vi "Append image and delete if possible.vi"(0 "report in":refnum<class "NI_Standard Report.lvclass">, 1 "alignment (default)":T1, 5 "path to image":path, 11 "error in (no error)":errorcluster, 12 "caption or alternative string":string, 13 "MS Office parameters":T2) -> (4 "report out":refnum<class "NI_Standard Report.lvclass">, 8 "start out (Word)":i32, 10 "end out (Word)":i32, 15 "error out":errorcluster)   [LabVIEW 2017, in "NI_Standard Report.lvclass"]
uses:
  <vilib>/Utility/NIReport.llb/Standard Report/NI_Standard Report.lvclass
  e:/builds/penguin/labview/branches/2017/dev/dist/vi.lib/Utility/NIReport.llb/NI_report.lvclass
  <vilib>/Utility/NIReport.llb/HTML Report Image Alignment.ctl
  <vilib>/Utility/NIReport.llb/NI_report.lvclass
  <vilib>/Utility/NIReport.llb/NI_ReportGenerationCore.lvlib
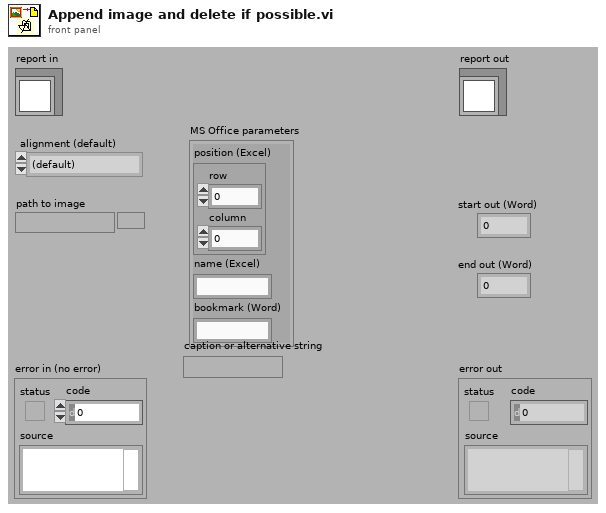
[diagram p1: front panel]
types:
  T1 = typedef "NI_ReportGenerationCore.lvlib/HTML Report Image Alignment.ctl" = enum16{"(default)", "LEFT", "RIGHT", "TOP", "TEXTTOP", "MIDDLE", "ABSMIDDLE", "BASELINE", "BOTTOM", "ABSBOTTOM"}
  T2 = cluster{"position (Excel)":cluster{"row":i32, "column":i32}, "name (Excel)":string, "bookmark (Word)":string}
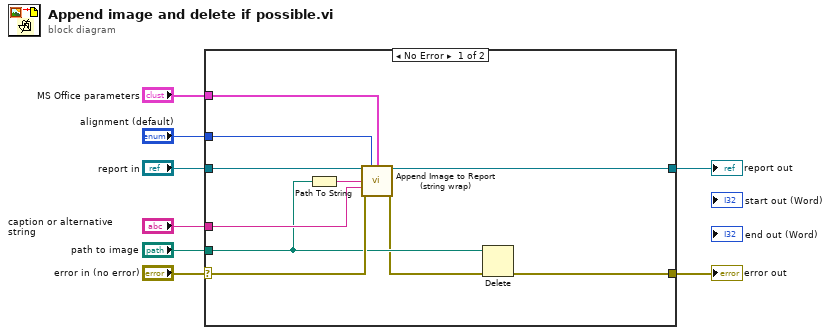
[diagram p0: block diagram]
diagram:
  n1 = case shown="No Error" "error in (no error)" {
    selector: "error in (no error)" -> [w17 w20]
    tunnel: [w9 w20] -> w7
    tunnel: [w10 w19] -> w5
    tunnel: "report in" -> [w11 w19]
    tunnel: "MS Office parameters" -> [w16 _]
    tunnel: "alignment (default)" -> [w15 _]
    tunnel: "caption or alternative string" -> [w14 _]
    tunnel: "path to image" -> [w13 _]
    frame No Error {
      n2 = Path To String(path=w13) -> (string=w18:string)
      n3 = call <vilib>:"Append Image to Report (string wrap).vi"("report in"=w11, "alignment (default)"=w15, "MS Office parameters"=w16, "path or URL of image"=w18, "caption or alternative string"=w14, "error in (no error)"=w17) -> ("report out"=w10:refnum<class "NI_Standard Report.lvclass">, "error out"=w12:errorcluster)  [unwired: 8 out]
      n4 = Delete(path (use dialog)=w13, error in=w12) -> (error out=w9:errorcluster)  [unwired: 5 out]
    }
    frame Error {
    }
  }
  "error out" <- w7
  "report out" <- w5
